vi "Check if Windows Service Exists.vi"(8 "error in (no error)":errorcluster, 11 "service name":string="NITaggerService") -> (0 "error out":errorcluster, 2 "service exist?":bool=TRUE, 3 "service name out":string="NITaggerService", 4 "console out":string="SERVICE_NAME: NITaggerService\r\nTRUE")   [LabVIEW 2017]
doc: "Checks whether a Windows service matching str is installed, by querying the service list through System Exec. Returns the matched service name and the raw console output."
uses:
  Configuration/Ini/ini_configuration.lvlib
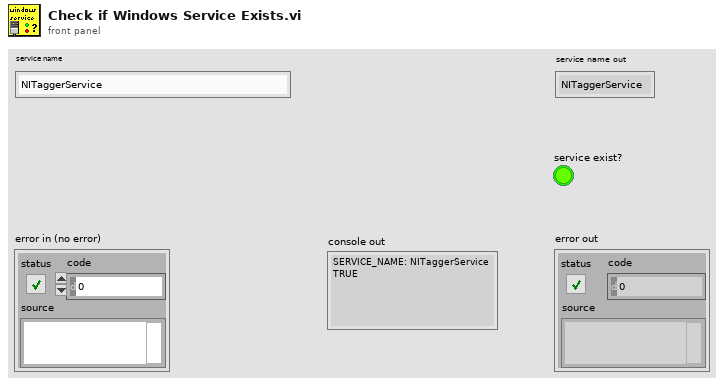
[diagram p1: front panel]
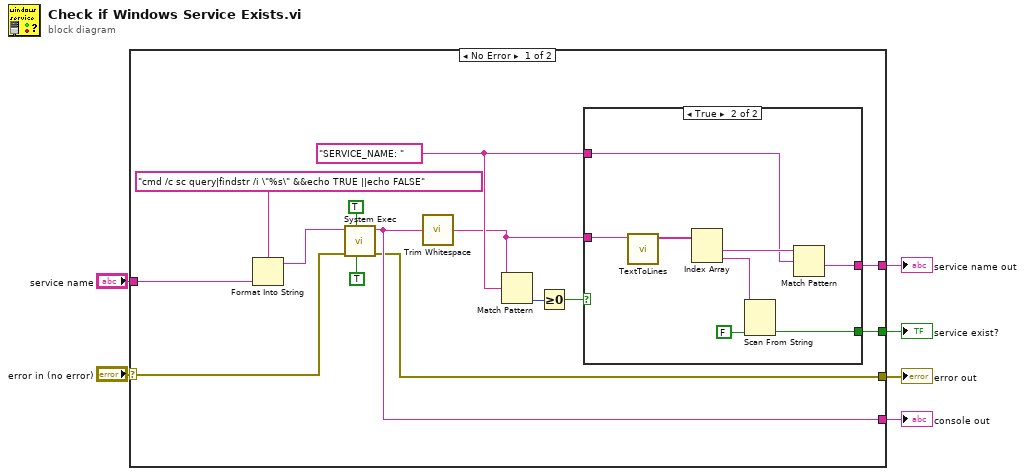
[diagram p0: block diagram]
diagram:
  n1 = case shown="No Error" "error in (no error)" {
    selector: "error in (no error)" -> [w8 w29]
    tunnel: [w18 _] -> w6
    tunnel: [w17 _] -> w5
    tunnel: "service name" -> [w14 _]
    tunnel: [w12 _] -> w3
    tunnel: [w7 w29] -> w1
    frame No Error {
      w13 = "SERVICE_NAME: " ("regular expression")
      n2 = Format Into String(format string="cmd /c sc query|findstr /i \"%s\" &&echo TRUE ||echo FALSE" ("command line"), w14) -> (resulting string=w15:string)  [unwired: 2 in, 1 out]
      n3 = call <vilib>:"System Exec.vi"("run minimized? (F)"=TRUE, "wait until completion? (T)"=TRUE, "error in (no error)"=w8, "command line"=w15) -> ("error out"=w7:errorcluster, "standard output"=w12:string)  [unwired: 4 in, 2 out]
      n4 = call <vilib>:"Trim Whitespace.vi"("string"=w12) -> ("trimmed string"=w11:string)  [unwired: 1 in]
      n5 = Match Pattern(string=w11, regular expression=w13) -> (offset past match=w10:i32)  [unwired: 1 in, 3 out]
      n6 = Greater Or Equal To 0?(x=w10) -> (x >= 0?=w9:bool)
      n7 = case shown="True" w9 {
        tunnel: [_ w25] -> w18
        tunnel: [_ w24] -> w17
        tunnel: w13 -> [_ w23]
        tunnel: w11 -> [_ w22]
        frame False {
        }
        frame True {
          n8 = call "TextToLines.vi"("string"=w22) -> ("Lines"=w21:string[])  [unwired: 9 in, 1 out]
          n9 = Index Array(array=w21) -> (element #1=w26:string, element #2=w28:string)  [unwired: 2 in]
          n10 = Scan From String(input string=w28, default 1=FALSE) -> (output 1=w24:bool)  [unwired: 3 in, 3 out]
          n11 = Match Pattern(string=w26, regular expression=w23) -> (after substring=w25:string)  [unwired: 1 in, 3 out]
        }
      }
    }
    frame Error {
    }
  }
  "console out" <- w3
  "service name out" <- w6
  "service exist?" <- w5
  "error out" <- w1
